vi "CreateClass.vi"(7 "PythonConverter_BD in":refnum<class "PyConvBD.lvclass">, 8 "error in":errorcluster, 11 "FlatSequenceFrame in":refnum<class "FlatSequenceFrame.lvclass">) -> (0 "error out":errorcluster, 3 "FlatSequenceFrame out":refnum<class "FlatSequenceFrame.lvclass">, 4 "class":string, 5 "PythonConverter_BD out":refnum<class "PyConvBD.lvclass">)   [LabVIEW 2014, in "FlatSequenceFrame.lvclass"]
uses:
  FlatSequenceFrame.lvclass
  Python/PythonConverter_BD/PyConvBD.lvclass
  FlatSequenceFrame.lvclass/FlatSequenceFrame.ctl
  Diagram/Diagram.lvclass
  Python/Parsing/Python Functions.lvlib
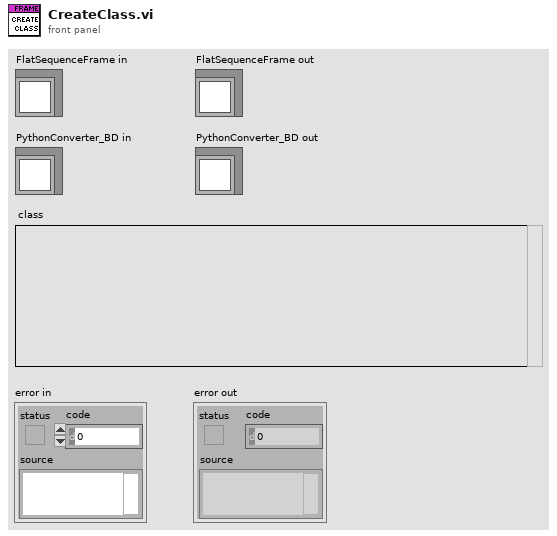
[diagram p1: front panel]
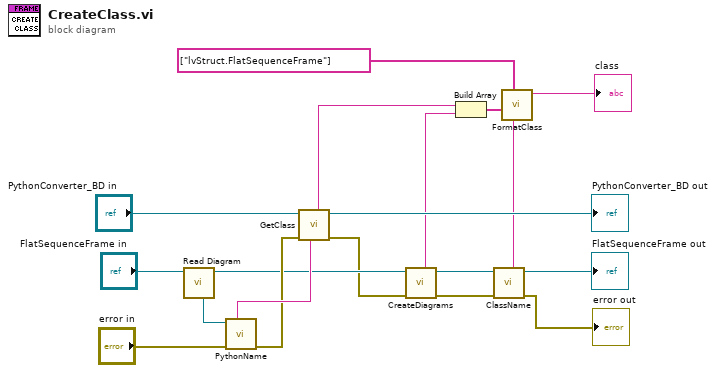
[diagram p0: block diagram]
diagram:
  n1 = call "Read Diagram.vi"("FlatSequenceFrame in"="FlatSequenceFrame in") -> ("FlatSequenceFrame out"=w6:refnum<class "FlatSequenceFrame.lvclass">, "Diagram"=w9:refnum<class "Diagram.lvclass">)  [unwired: 7 in]
  n2 = call-dynamic "PythonName.vi"("error in"="error in", "Diagram in"=w9) -> ("error out"=w17:errorcluster, "UID"=w18:string)  [unwired: 6 in, 2 out]
  n3 = call "GetClass.vi"("name"=w18, "error in"=w17, "PythonConverter_BD in"="PythonConverter_BD in") -> ("error out"=w5:errorcluster, "PythonConverter_BD out"=→"PythonConverter_BD out":refnum<class "PyConvBD.lvclass">, "class"=w10:string)  [unwired: 4 in]
  n4 = call-dynamic "CreateDiagrams.vi"("error in"=w5, "Structure in"=w6) -> ("error out"=w4:errorcluster, "Structure out"=w3:refnum<class "FlatSequenceFrame.lvclass">, "create_diagrams"=w2:string)  [unwired: 5 in]
  n5 = Build Array(w10, w2) -> (w11:string[])
  n6 = call-dynamic "ClassName.vi"("error in"=w4, "FlatSequenceFrame in"=w3) -> ("error out"=→"error out":errorcluster, "FlatSequenceFrame out"=→"FlatSequenceFrame out":refnum<class "FlatSequenceFrame.lvclass">, "name"=w1:string)  [unwired: 6 in, 1 out]
  n7 = call "FormatClass.vi"("name"=w1, "parameters/ancestors"=string[] ["lvStruct.FlatSequenceFrame"], "body"=w11) -> ("python"=→"class":string)  [unwired: 8 in]
